vi "Get_LEM_Response.vi"(6 "Hratio":dbl, 8 "Cavity Pressure Magnitude":dbl, 9 "Cavity Pressure Phase":dbl, 10 "Fluid Properties":T1={"R"=8.31451, "Mair"=0.0289645, "T"=293.0, "Patmos"=101325.0, "gamma"=1.4}, 11 "SJ Data IN":T2) -> (0 "Phi":dbl, 1 "Phi*":dbl, 2 "Uo":dbl, 3 "U*":dbl, 4 "OmegaH":dbl)   [LabVIEW 2011]
uses:
  Controls/SJ_Data_Cluster.ctl
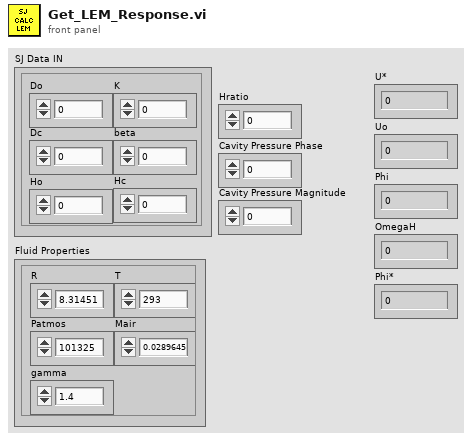
[diagram p1: front panel]
types:
  T1 = cluster{"R":dbl, "Mair":dbl, "T":dbl, "Patmos":dbl, "gamma":dbl}
  T2 = typedef "SJ_Data_Cluster.ctl" = cluster{"Do":dbl, "Dc":dbl, "Ho":dbl, "Hc":dbl, "K":dbl, "beta":dbl}
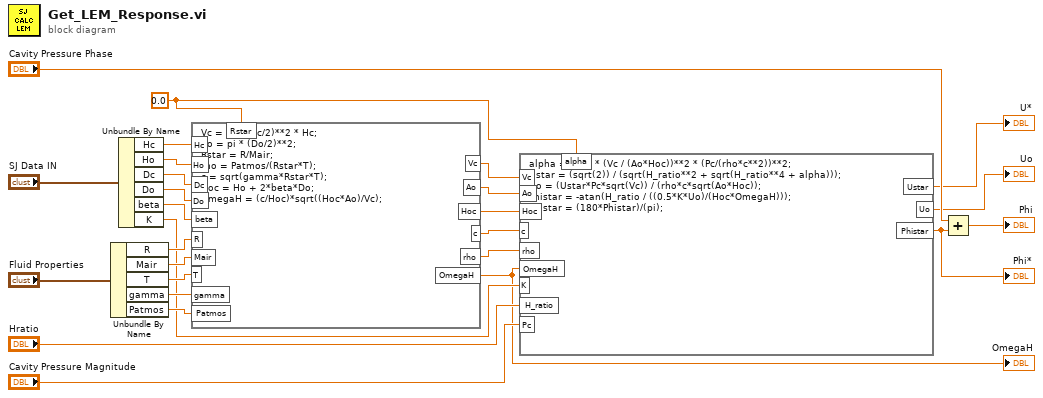
[diagram p0: block diagram]
diagram:
  w1 = 0.0 ("input variable")
  n1 = Unbundle By Name("Fluid Properties") -> ("R"=w22:dbl, "Mair"=w21:dbl, "T"=w20:dbl, "gamma"=w19:dbl, "Patmos"=w18:dbl)
  n2 = Unbundle By Name("SJ Data IN") -> ("Hc"=w27:dbl, "Ho"=w26:dbl, "Dc"=w25:dbl, "Do"=w24:dbl, "beta"=w10:dbl, "K"=w9:dbl)
  n3 = formula code="Vc = pi * (Dc/2)**2 * Hc; \nAo = pi * (Do/2)**2;\nRstar = R/Mair; \nrho = Patmos/(Rstar*T);\nc = sqrt(gamma*Rstar*T); \nHoc = Ho + 2*beta*Do; \nOmegaH = (c/Hoc)*sqrt((Hoc*Ao)/Vc);"("Do"=w24, "R"=w22, "Mair"=w21, "T"=w20, "gamma"=w19, "Ho"=w26, "Dc"=w25, "Hc"=w27, "Patmos"=w18, "beta"=w10, "Rstar"=w1) -> ("Vc"=w17:dbl, "Ao"=w16:dbl, "Hoc"=w15:dbl, "c"=w14:dbl, "rho"=w13:dbl, "OmegaH"=w7:dbl)
  "OmegaH" <- w7
  n4 = formula code="alpha = K**2 * (Vc / (Ao*Hoc))**2 * (Pc/(rho*c**2))**2;\nUstar = (sqrt(2)) / (sqrt(H_ratio**2 + sqrt(H_ratio**4 + alpha)));\nUo = (Ustar*Pc*sqrt(Vc)) / (rho*c*sqrt(Ao*Hoc));\nPhistar = -atan(H_ratio / ((0.5*K*Uo)/(Hoc*OmegaH)));\nPhistar = (180*Phistar)/(pi);"("c"=w14, "rho"=w13, "OmegaH"=w7, "K"=w9, "H_ratio"="Hratio", "Ao"=w16, "Hoc"=w15, "Vc"=w17, "Pc"="Cavity Pressure Magnitude", "alpha"=w1) -> ("Ustar"=→"U*":dbl, "Uo"=→"Uo":dbl, "Phistar"=w5:dbl)
  "Phi*" <- w5
  n5 = Add(x="Cavity Pressure Phase", y=w5) -> (x+y=→"Phi":dbl)
